vi "Signal Bank.vi"(1 "Action":enum16{"Add", "Replace ID", "Read ID", "Clear"}(ring), 7 "1D Data In":dbl[](array[numeric]) format="%.2f", 11 "ID":string) -> (3 "Found?":bool, 8 "1D Data Out":dbl[](array[numeric]))   [LabVIEW 2020]
uses:
  Utility VIs/Array Dimensions (2D).vi
panel:
  out "Nsignals":i32
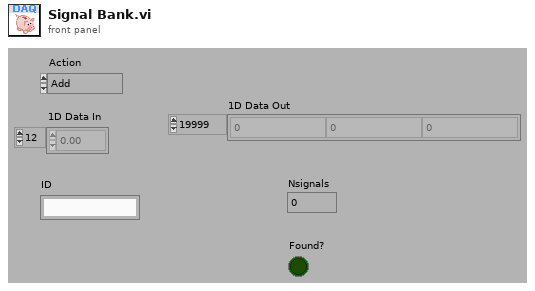
[diagram p1: front panel]
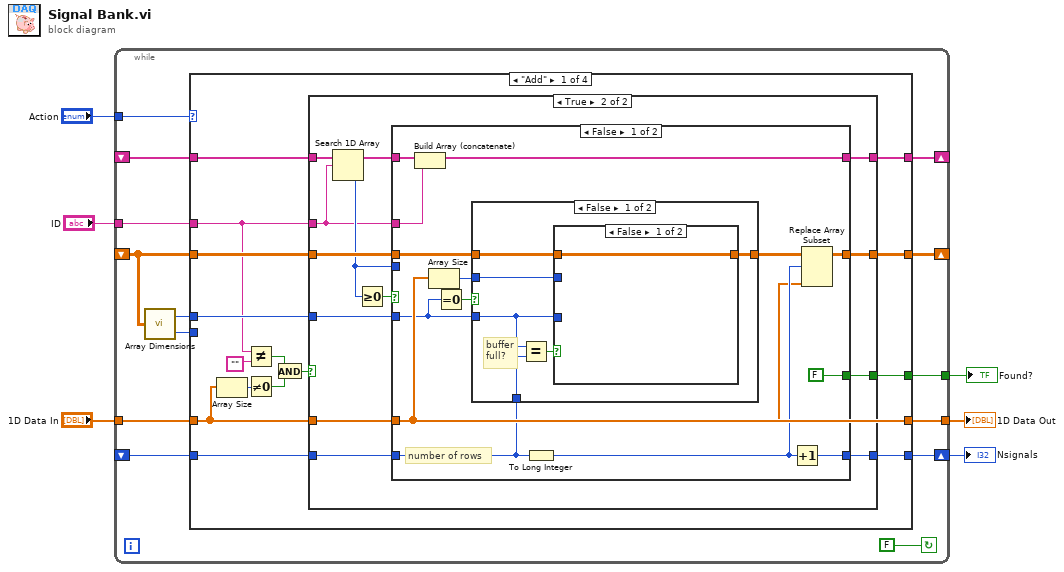
[diagram p0: block diagram]
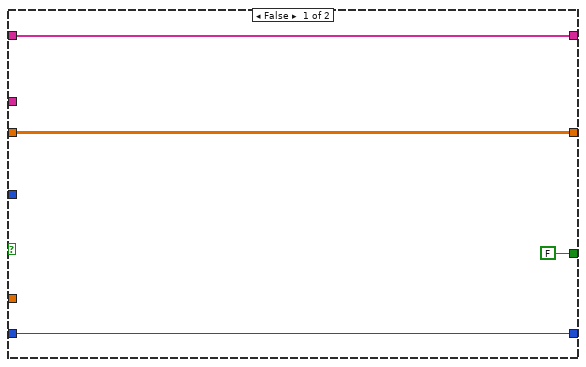
[diagram p2: hidden frame]
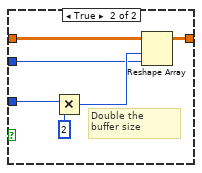
[diagram p3: hidden frame]
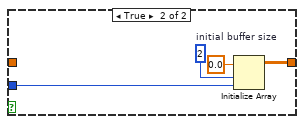
[diagram p4: hidden frame]
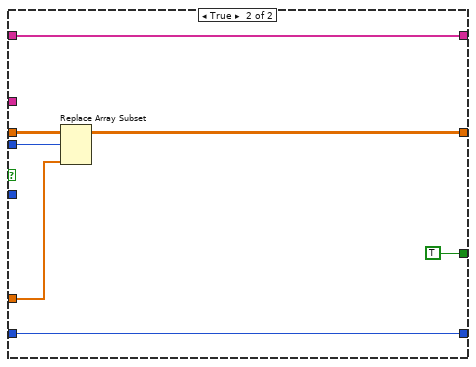
[diagram p5: hidden frame]
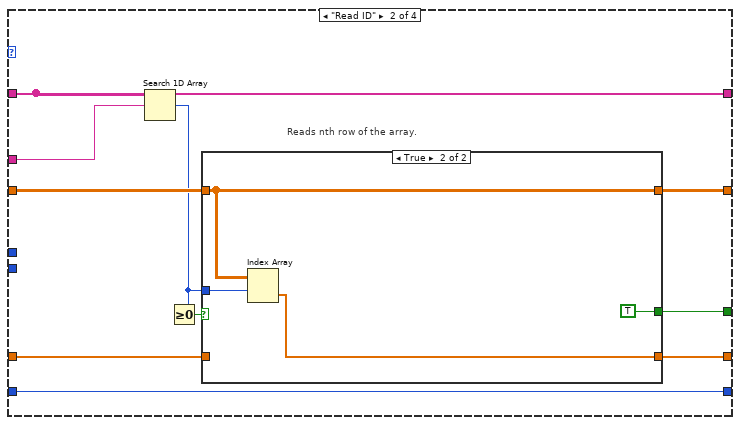
[diagram p6: hidden frame]
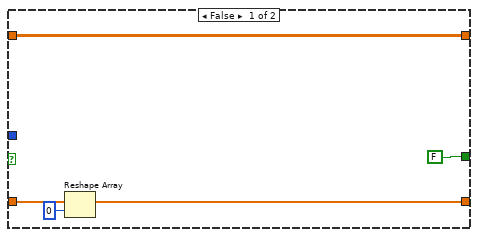
[diagram p7: hidden frame]
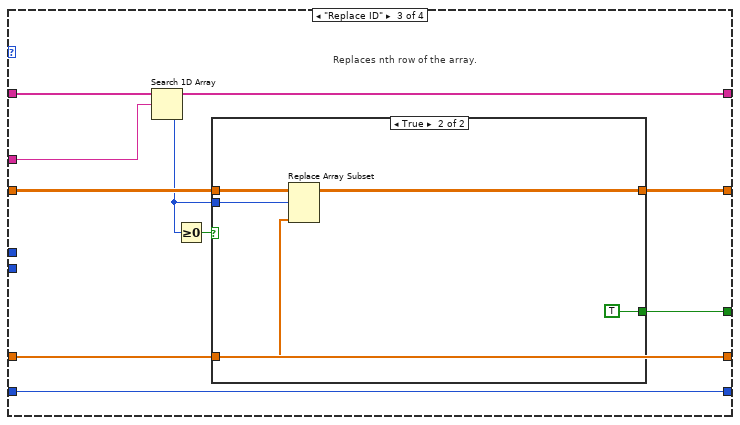
[diagram p8: hidden frame]
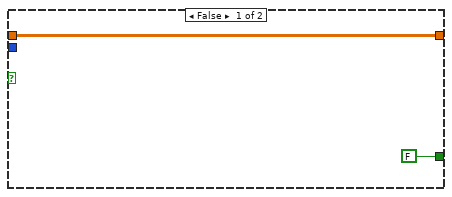
[diagram p9: hidden frame]
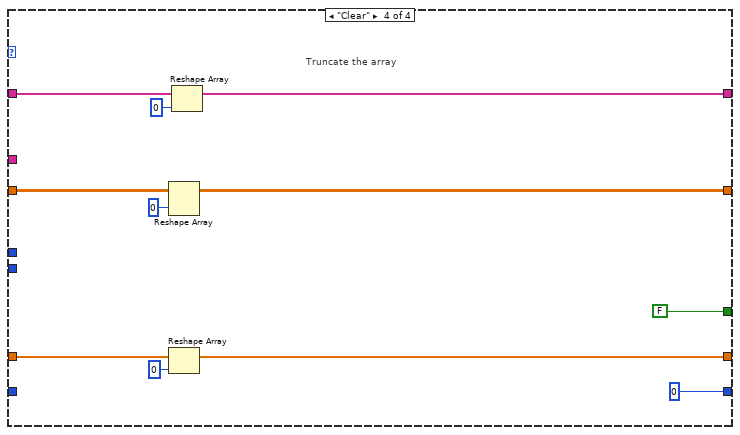
[diagram p10: hidden frame]
diagram:
  n1 = while {
    tunnel: "1D Data In" -> [w16]
    shift-left: _ -> [w18]
    shift-right: [w17] -> w3
    shift-left: _ -> [w15]
    shift-right: [w19] -> _
    tunnel: "Action" -> [w20]
    tunnel: [w11] -> w1
    tunnel: "ID" -> [w10]
    shift-right: [w9] -> _
    shift-left: _ -> [w8]
    tunnel: [w7] -> w2
    stop <- FALSE continue-if-true
    n2 = call-poly "Array Dimensions.vi"("2D Array"=w15) -> ("# rows"=w14:i32, "# columns"=w13:i32)  [unwired: 13 in]
    n3 = case shown="\"Add\"" w20 {
      tunnel: w15 -> [w32 w98 w116 w135]
      tunnel: [w35 w97 w115 w134] -> w19
      tunnel: w18 -> [w33 w93 w117 _]
      tunnel: [w34 w93 w117 0] -> w17
      tunnel: w16 -> [w27 w96 w110 w131]
      tunnel: w14 -> [w31 _ _ _]
      tunnel: w13 -> [_ _ _ _]
      tunnel: [w27 w95 w110 w130] -> w11
      tunnel: w10 -> [w21 w94 w114 _]
      tunnel: [w30 w92 w111 w127] -> w9
      tunnel: w8 -> [w29 w92 w111 w128]
      tunnel: [w28 w91 w109 FALSE] -> w7
      frame "Add" {
        n4 = Array Size(array=w27) -> (size(s)=w25:i32)
        n5 = Not Equal?(x=w21, y="") -> (x != y?=w23:bool)
        n6 = Not Equal To 0?(x=w25) -> (x != 0?=w24:bool)
        n7 = And(x=w23, y=w24) -> (x .and. y?=w26:bool)
        n8 = case shown="True" w26 {
          tunnel: [w38 w51] -> w35
          tunnel: [w39 w50] -> w34
          tunnel: w33 -> [w39 w49]
          tunnel: w32 -> [w38 w48]
          tunnel: w31 -> [_ w47]
          tunnel: w27 -> [_ w46]
          tunnel: [w37 w45] -> w30
          tunnel: w29 -> [w37 w44]
          tunnel: w21 -> [_ w41]
          tunnel: [FALSE w40] -> w28
          frame False {
          }
          frame True {
            n9 = Search 1D Array(1D array=w44, element=w41) -> (index of element=w42:i32)  [unwired: 1 in]
            n10 = Greater Or Equal To 0?(x=w42) -> (x >= 0?=w43:bool)
            n11 = case shown="False" w43 {
              tunnel: [w58 w86] -> w51
              tunnel: [w65 w89] -> w50
              tunnel: w49 -> [w64 w89]
              tunnel: w48 -> [w63 w87]
              tunnel: w47 -> [w52 _]
              tunnel: w46 -> [w55 w85]
              tunnel: w41 -> [w62 _]
              tunnel: [w61 w88] -> w45
              tunnel: w44 -> [w60 w88]
              tunnel: w42 -> [_ w84]
              tunnel: [FALSE TRUE] -> w40
              frame False {
                # "number of rows"
                n12 = Build Array (concatenate)(w60, w62) -> (w61:string[])
                n13 = Array Size(array=w55) -> (size(s)=w54:i32)
                n14 = Equal To 0?(x=w52) -> (x = 0?=w53:bool)
                n15 = case shown="False" w53 {
                  tunnel: w64 -> [w71 _]
                  tunnel: w63 -> [w70 _]
                  tunnel: w52 -> [w69 _]
                  tunnel: [w67 w79] -> w59
                  tunnel: w54 -> [w66 w80]
                  frame False {
                    # "buffer\nfull?"
                    n16 = Equal?(x=w69, y=w71) -> (x = y?=w68:bool)
                    n17 = case shown="False" w68 {
                      tunnel: w70 -> [w72 w75]
                      tunnel: [w72 w76] -> w67
                      tunnel: w69 -> [_ w74]
                      tunnel: w66 -> [_ w73]
                      frame False {
                      }
                      frame True {
                        # "Double the\nbuffer size"
                        n18 = Multiply(x=w74, y=2) -> (x*y=w77:i32)
                        n19 = Reshape Array(w75, w77, w73) -> (w76:dbl[][])
                      }
                    }
                  }
                  frame True {
                    w81 = 2  # initial buffer size
                    n20 = Initialize Array(0.0 ("element"), w81, w80) -> (w79:dbl[][])
                  }
                }
                n21 = To Long Integer(number=w64) -> (32bit integer=w57:i32)
                n22 = Increment(x=w57) -> (x+1=w65:i32)
                n23 = Replace Array Subset(array=w59, new element=w55, index (row)=w57) -> (w58:dbl[][])  [unwired: 1 in]
              }
              frame True {
                n24 = Replace Array Subset(array=w87, new element=w85, index (row)=w84) -> (w86:dbl[][])  [unwired: 1 in]
              }
            }
          }
        }
      }
      frame "Read ID" {
        # "Reads nth row of the array."
        n25 = Search 1D Array(1D array=w92, element=w94) -> (index of element=w90:i32)  [unwired: 1 in]
        n26 = Greater Or Equal To 0?(x=w90) -> (x >= 0?=w99:bool)
        n27 = case shown="True" w99 {
          tunnel: w98 -> [w104 w107]
          tunnel: [w104 w107] -> w97
          tunnel: w96 -> [w103 _]
          tunnel: [w102 w108] -> w95
          tunnel: w90 -> [_ w106]
          tunnel: [FALSE TRUE] -> w91
          frame False {
            n28 = Reshape Array(w103, 0 ("dimension size")) -> (w102:dbl[])
          }
          frame True {
            n29 = Index Array(array=w107, index (row)=w106) -> (element=w108:dbl[])  [unwired: 1 in]
          }
        }
      }
      frame "Replace ID" {
        # "Replaces nth row of the array."
        n30 = Search 1D Array(1D array=w111, element=w114) -> (index of element=w112:i32)  [unwired: 1 in]
        n31 = Greater Or Equal To 0?(x=w112) -> (x >= 0?=w113:bool)
        n32 = case shown="True" w113 {
          tunnel: w116 -> [w119 w124]
          tunnel: [w119 w123] -> w115
          tunnel: w112 -> [_ w121]
          tunnel: w110 -> [_ w122]
          tunnel: [FALSE TRUE] -> w109
          frame False {
          }
          frame True {
            n33 = Replace Array Subset(array=w124, new element=w122, index (row)=w121) -> (w123:dbl[][])  [unwired: 1 in]
          }
        }
      }
      frame "Clear" {
        w132 = 0
        # "Truncate the array"
        n34 = Reshape Array(w135, w132, w132) -> (w134:dbl[][])
        n35 = Reshape Array(w131, 0 ("dimension size")) -> (w130:dbl[])
        n36 = Reshape Array(w128, 0 ("dimension size")) -> (w127:string[])
      }
    }
  }
  "1D Data Out" <- w1
  "Nsignals" <- w3
  "Found?" <- w2
